vi "dfd_CIC Moving Average Simu.vi"(0 "signal in":i32[](array[numeric]), 3 "init? (T)":bool, 5 "factor":i32, 9 "Output MSB pos":i16, 11 "FXPMRateSimState in":T1, 12 "Output wl":i16, 13 "q_mode":T3=enum."Truncation" caption="rounding mode") -> (4 "signal out":i32[](array[numeric]) format="%.0x", 15 "FXPMRateSimState out":T1)   [LabVIEW 2017, in "NI_DigFilter_FXP.lvlib"]
uses:
  <vilib>/addons/Digital Filter Design/NI_DigFilter_FXP.lvlib
  <vilib>/addons/Digital Filter Design/_Objects.llb/DFD Round-off Mode.ctl
  <vilib>/addons/Digital Filter Design/_Objects.llb/dfd_FXP MRate Simu State.ctl
  <vilib>/addons/Digital Filter Design/_Objects.llb/dfd_Integer I160.ctl
  <vilib>/addons/Digital Filter Design/NI_DigFilterLicensed.lvlib
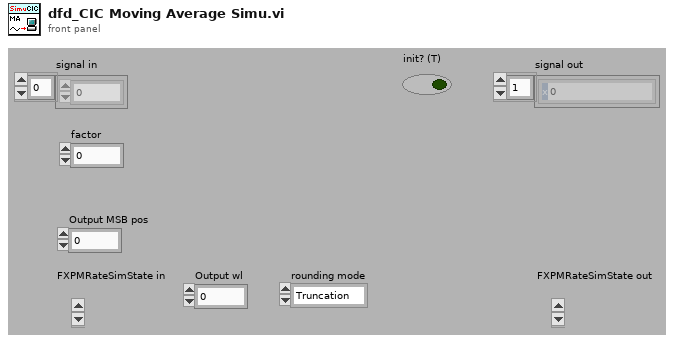
[diagram p1: front panel]
types:
  T1 = typedef "dfd_FXP MRate Simu State.ctl" = cluster{"acc1":T2[], "acc2":T2[], "FIR state":i64[], "next phase":i32}
  T2 = typedef "dfd_Integer I160.ctl" = cluster{"Hi [I32]":i32, "Lo3 [U32]":u32, "Lo2 [U32]":u32, "Lo1 [U32]":u32, "Lo0 [U32]":u32}
  T3 = typedef "NI_DigFilterLicensed.lvlib/DFD Round-off Mode.ctl" = enum16{"Nearest", "Truncation"}
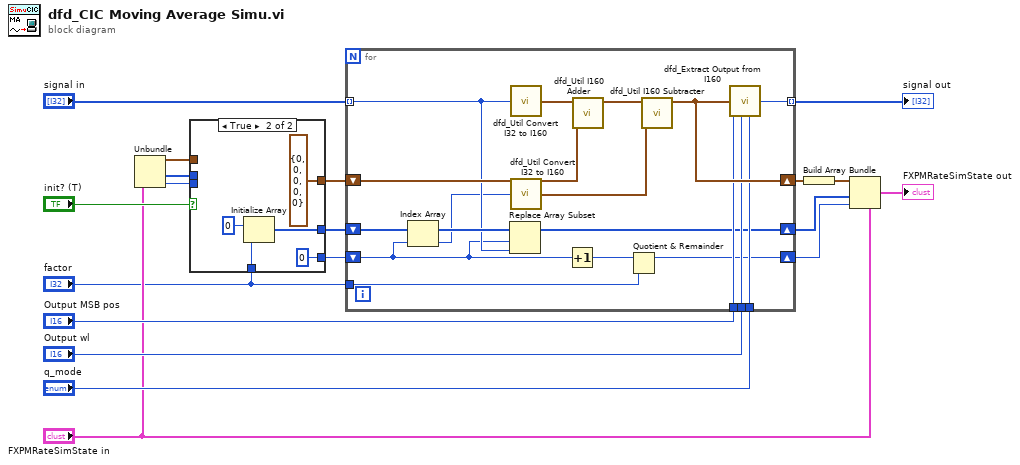
[diagram p0: block diagram]
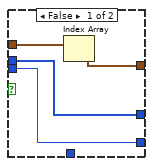
[diagram p2: hidden frame]
diagram:
  n1 = Unbundle("FXPMRateSimState in") -> ("acc1"=w18:T2[], "FIR state"=w17:i64[], "next phase"=w16:i32)  [unwired: 1 out]
  n2 = case shown="True" "init? (T)" {
    tunnel: w18 -> [w23 _]
    tunnel: w17 -> [w21 _]
    tunnel: w16 -> [w20 _]
    tunnel: [w22 T2 {"Hi [I32]"=0, "Lo3 [U32]"=0, "Lo2 [U32]"=0, "Lo1 [U32]"=0, "Lo0 [U32]"=0} ("x [I160]")] -> w15
    tunnel: "factor" -> [_ w26]
    tunnel: [w21 w25] -> w14
    tunnel: [w20 0 ("element")] -> w13
    frame False {
      n3 = Index Array(array=w23) -> (element=w22:T2)  [unwired: 1 in]
    }
    frame True {
      n4 = Initialize Array(0 ("element"), w26) -> (w25:i32[])
    }
  }
  n5 = for {
    shift-right: [w37] -> w6
    shift-left: w15 -> [w44]
    shift-right: [w32] -> w4
    shift-left: w14 -> [w43]
    shift-right: [w29] -> w3
    shift-left: w13 -> [w38]
    tunnel: "signal in" -> [w42] mode=indexing
    tunnel: "Output MSB pos" -> [w36]
    tunnel: "Output wl" -> [w35]
    tunnel: "q_mode" -> [w34]
    tunnel: [w33] -> w8 mode=indexing
    tunnel: "factor" -> [w30]
    n6 = Index Array(array=w43, index=w38) -> (element=w41:i64)
    n7 = Replace Array Subset(array=w43, new element=w42, index=w38) -> (w32:i64[])
    n8 = call <vilib>:"dfd_Util Convert I32 to I160.vi"("x [I32]"=w42) -> ("x [I160]"=w45:T2)  [unwired: 8 out]
    n9 = call <vilib>:"dfd_Util Convert I32 to I160.vi"("x [I32]"=w41) -> ("x [I160]"=w39:T2)  [unwired: 8 out]
    n10 = Increment(x=w38) -> (x+1=w31:i32)
    n11 = call <vilib>:"dfd_Util I160 Adder.vi"("y160"=w44, "x160"=w45) -> ("x+y160"=w40:T2)  [unwired: 9 out]
    n12 = Quotient & Remainder(x=w31, y=w30) -> (x-y*floor(x/y)=w29:i32)  [unwired: 1 out]
    n13 = call <vilib>:"dfd_Util I160 Subtracter.vi"("y [I160]"=w39, "x [I160]"=w40) -> ("x-y [I160]"=w37:T2)  [unwired: 9 out]
    n14 = call <vilib>:"dfd_Extract Output from I160.vi"("I160"=w37, "output MSB pos"=w36, "Output wl"=w35, "q_mode"=w34) -> ("y"=w33:i32)  [unwired: 5 out]
  }
  "signal out" <- w8
  n15 = Build Array(w6) -> (w5:T2[])
  n16 = Bundle(cluster="FXPMRateSimState in", "acc1"=w5, "FIR state"=w4, "next phase"=w3) -> (→"FXPMRateSimState out":T1)  [unwired: 1 out]
